vi "GettingHistoricalDataA.vi"() -> ()   [LabVIEW 2020]
uses:
  StateH.ctl
  Data2.ctl
  <vilib>/Utility/file.llb/Read Delimited Spreadsheet (DBL).vi
panel:
  out "StateH":T1=enum."Wait"
  in  "Open Button":bool
  in  "stop":bool
  in  "Play Button":bool
  out "Temperature Graph":T2(graph)
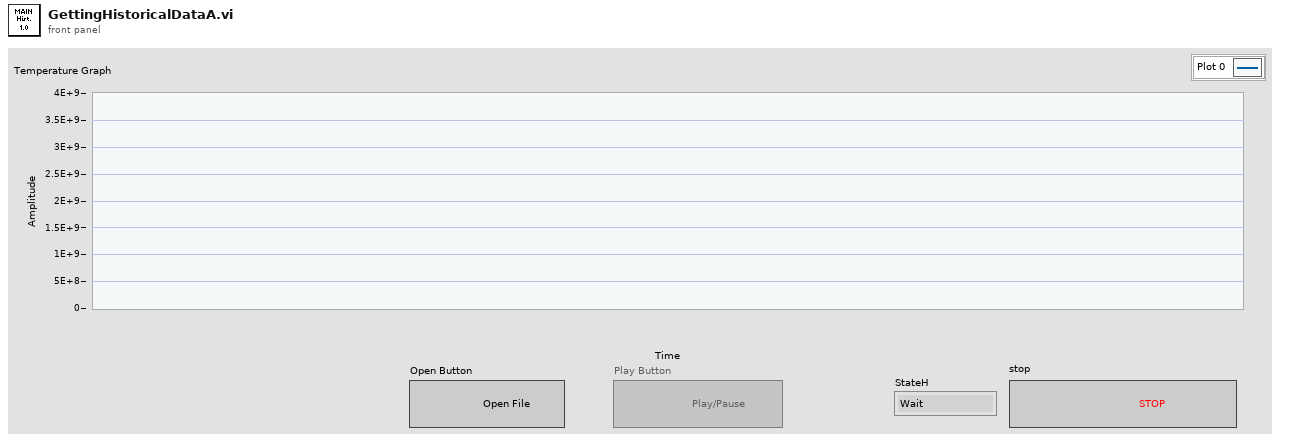
[diagram p1: front panel]
types:
  T1 = typedef "StateH.ctl" = enum16{"Initialize", "Wait", "OpenData", "Play", "Pause", "Finalize"}
  T2 = cluster{"seconds since 1Jan1904":timestamp, dbl, dbl}[]
  T3 = enum8{"Enabled", "Disabled", "Disabled and Grayed Out"}
  T4 = typedef "Data2.ctl" = cluster{"time":timestamp, "Temperature":dbl, "Viscosity":dbl}
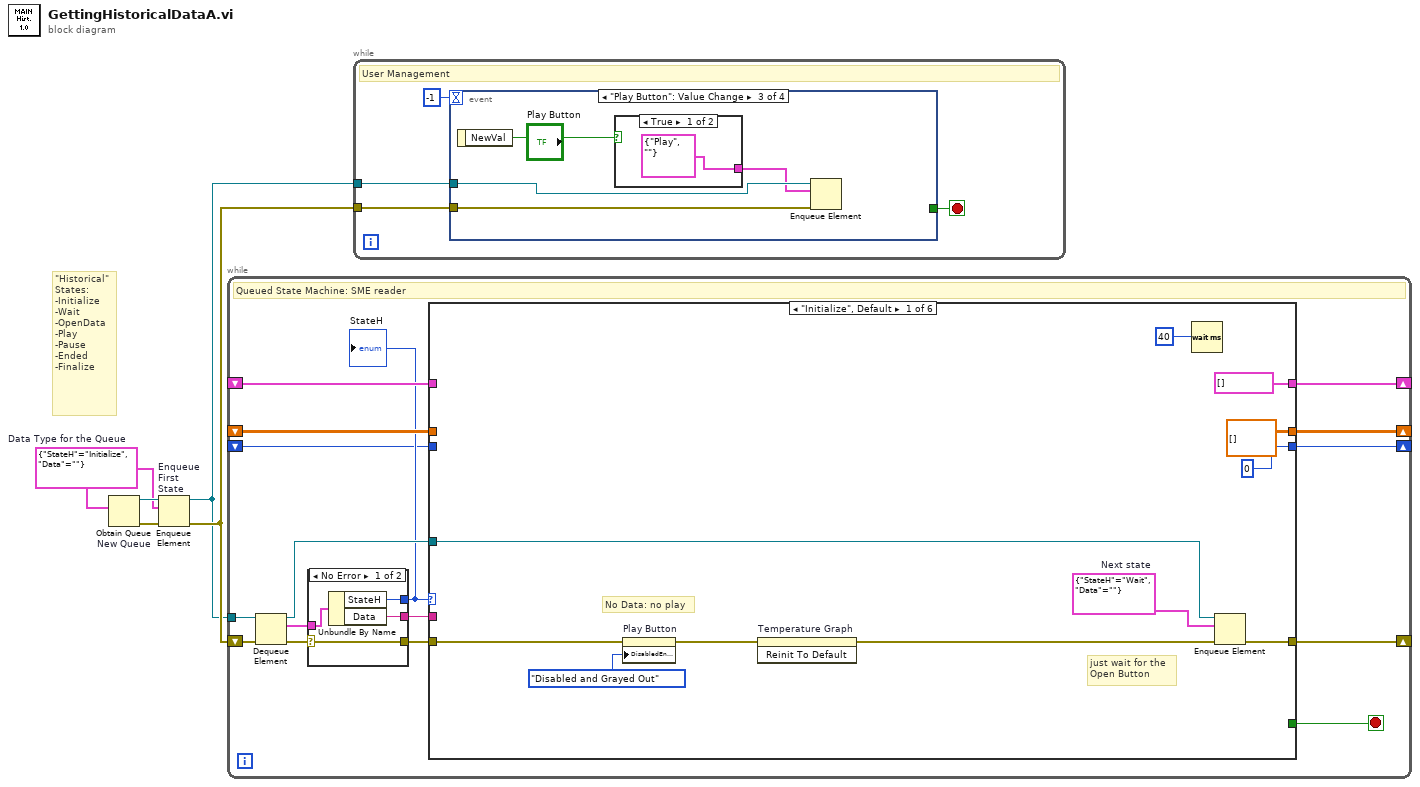
[diagram p0: block diagram]
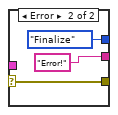
[diagram p2: hidden frame]
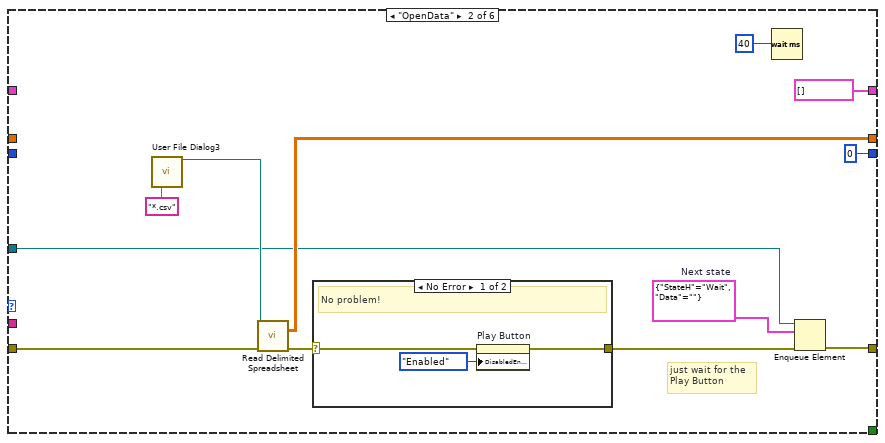
[diagram p3: hidden frame]
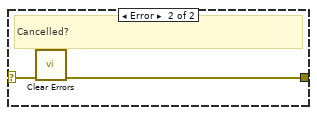
[diagram p4: hidden frame]
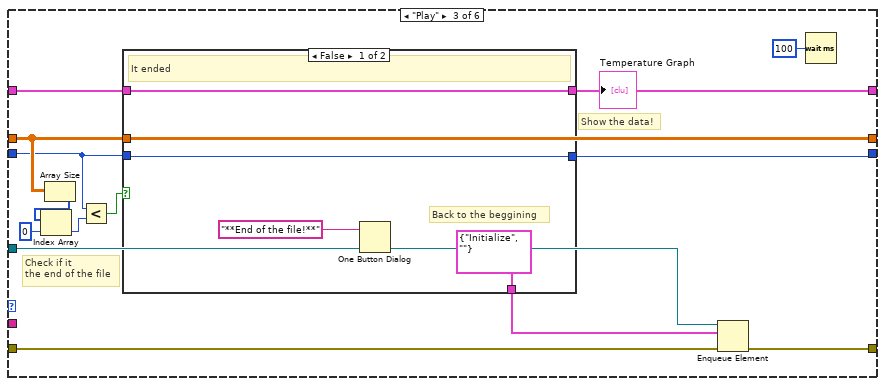
[diagram p5: hidden frame]
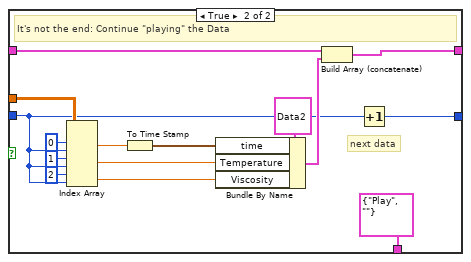
[diagram p6: hidden frame]
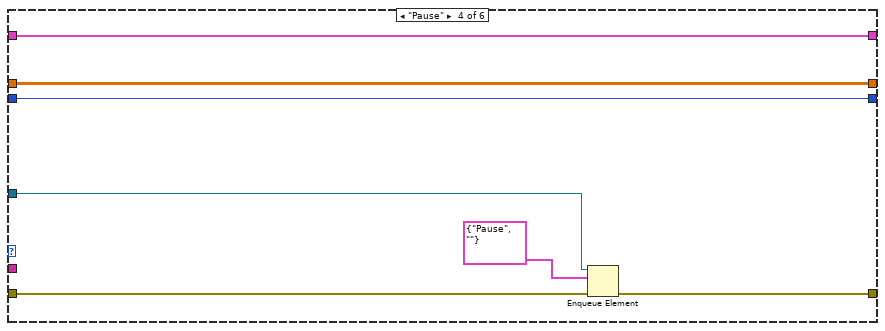
[diagram p7: hidden frame]
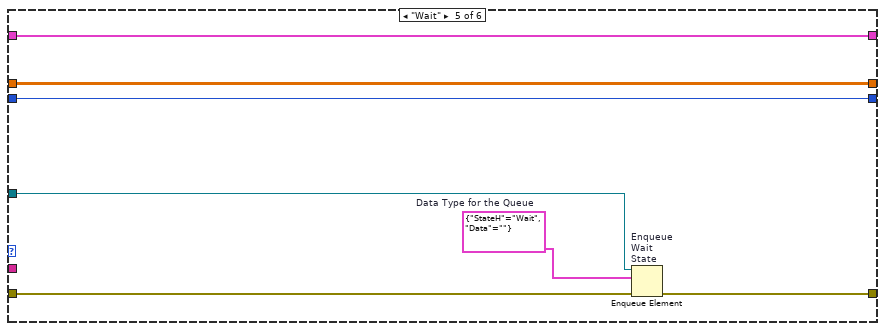
[diagram p8: hidden frame]
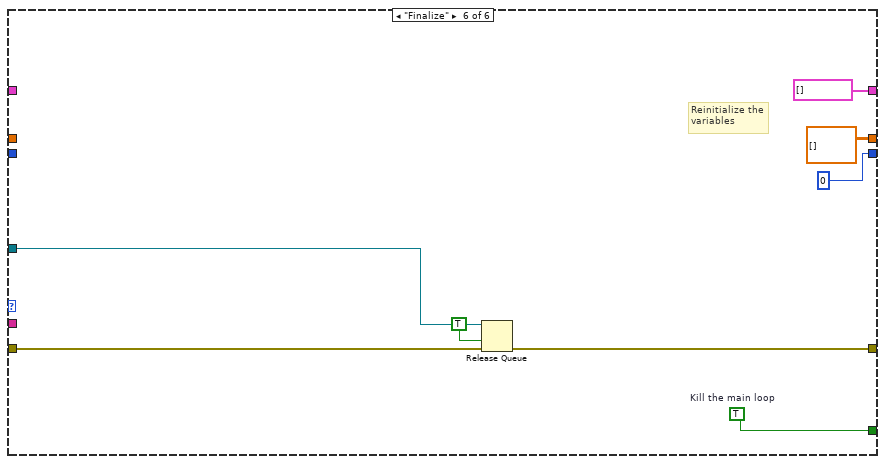
[diagram p9: hidden frame]
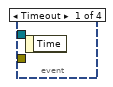
[diagram p10: hidden frame]
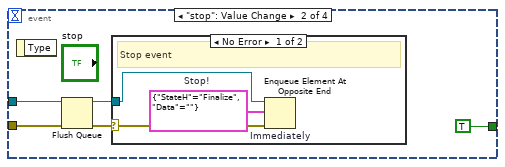
[diagram p11: hidden frame]
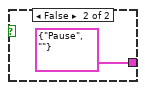
[diagram p13: hidden frame]
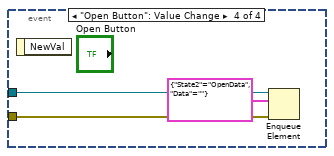
[diagram p14: hidden frame]
diagram:
  w4 = cluster{"StateH":T1, "Data":string} {"StateH"=enum."Initialize", "Data"=""}  # Data Type for the Queue
  # "\"Historical\"\nStates:\n-Initialize\n-Wait\n-OpenData\n-Play\n-Pause\n-Ended\n-Finalize"
  n1 = Obtain Queue "New Queue"(element data type=w4) -> (queue out=w5:refnum<queue>, error out=w3:errorcluster)  [unwired: 4 in, 1 out]
  n2 = Enqueue Element "Enqueue\nFirst\nState"(queue=w5, element=w4, error in (no error)=w3) -> (queue out=w1:refnum<queue>, error out=w2:errorcluster)  [unwired: 1 in, 1 out]
  n3 = while {
    shift-right: [w19] -> _
    shift-left: w2 -> [w18]
    shift-right: [w12] -> _
    shift-left: _ -> [w13]
    shift-right: [w11] -> _
    shift-left: _ -> [w10]
    tunnel: w1 -> [w9]
    shift-right: [w6] -> _
    shift-left: _ -> [w7]
    stop <- w15 stop-if-true
    # "Queued State Machine: SME reader"
    n4 = Dequeue Element(queue=w9, error in (no error)=w18) -> (queue out=w14:refnum<queue>, element=w16:cluster{"StateH":T1, "Data":string}, error out=w17:errorcluster)  [unwired: 1 in, 1 out]
    n5 = case shown="No Error" w17 {
      selector: w17 -> [w22 w27]
      tunnel: w16 -> [w25 _]
      tunnel: [w24 StateH."Finalize" ("StateH")] -> w8
      tunnel: [w23 "Error!" ("Data")] -> w21
      tunnel: [w22 w27] -> w20
      frame No Error {
        n6 = Unbundle By Name(w25) -> ("StateH"=w24:T1, "Data"=w23:string)
      }
      frame Error {
      }
    }
    "StateH" <- w8
    n7 = case shown="\"Initialize\", Default" w8 {
      tunnel: w21 -> [_ _ _ _ _ _]
      tunnel: w20 -> [w33 w41 w67 w90 w99 w106]
      tunnel: [w35 w42 w65 w91 w98 w110] -> w19
      tunnel: [_ _ _ _ _ w111] -> w15
      tunnel: w14 -> [w37 w45 w66 w92 w101 w109]
      tunnel: w13 -> [_ _ w69 w94 w103 _]
      tunnel: [T2 [] T2 [] w68 w94 w103 T2 []] -> w12
      tunnel: [dbl[][] [] ("all rows") w46 w63 w95 w102 dbl[][] [] ("all rows")] -> w11
      tunnel: w10 -> [_ _ w63 w95 w102 _]
      tunnel: w7 -> [_ _ w62 w96 w97 _]
      tunnel: [0 0 w64 w96 w97 0] -> w6
      frame "Initialize", Default {
        w36 = cluster{"StateH":T1, "Data":string} {"StateH"=enum."Wait", "Data"=""}  # Next state
        # "No Data: no play"
        # "just wait for the \nOpen Button"
        n8 = property on="Play Button" class="Bool"(error in=w33, "DisabledEnum"=T3."Disabled and Grayed Out" ("Disabled")) -> (error out=w30:errorcluster)  [unwired: 1 in, 1 out]
        n9 = invoke on="Temperature Graph" class="XYGraph (strict)" method="Reinit To Default"(error in=w30) -> (error out=w29:errorcluster)  [unwired: 2 in, 2 out]
        n10 = Wait (ms)(milliseconds to wait=u32 40) -> ()  [unwired: 1 out]
        n11 = Enqueue Element(queue=w37, element=w36, error in (no error)=w29) -> (error out=w35:errorcluster)  [unwired: 1 in, 2 out]
      }
      frame "OpenData" {
        w44 = cluster{"StateH":T1, "Data":string} {"StateH"=enum."Wait", "Data"=""}  # Next state
        # "just wait for the \nPlay Button"
        n12 = call "User File Dialog3"("pattern (all files)"="*.csv") -> ("selected path"=w47:path)  [unwired: 11 in, 3 out]
        n13 = call-poly <vilib>:"Read Delimited Spreadsheet.vi"("file path (dialog if empty)"=w47, "error in (no error)"=w41) -> ("all rows"=w46:dbl[][], "error out"=w49:errorcluster)  [unwired: 8 in, 4 out]
        n14 = case shown="No Error" w49 {
          selector: w49 -> [w54 w56]
          tunnel: [w53 w55] -> w43
          frame No Error {
            # "No problem!"
            n15 = property on="Play Button" class="Bool"(error in=w54, "DisabledEnum"=T3."Enabled" ("Disabled")) -> (error out=w53:errorcluster)  [unwired: 1 in, 1 out]
          }
          frame Error {
            # "Cancelled?"
            n16 = call <vilib>:"Clear Errors.vi"("error in (no error)"=w56) -> ("error out"=w55:errorcluster)  [unwired: 5 in, 1 out]
          }
        }
        n17 = Wait (ms)(milliseconds to wait=u32 40) -> ()  [unwired: 1 out]
        n18 = Enqueue Element(queue=w45, element=w44, error in (no error)=w43) -> (error out=w42:errorcluster)  [unwired: 1 in, 2 out]
      }
      frame "Play" {
        # "Check if it\nthe end of the file"
        # "Show the data!"
        n19 = Array Size(array=w63) -> (size(s)=w61:i32[])
        n20 = Index Array(array=w61, index=0) -> (element=w59:i32)
        n21 = Less?(x=w62, y=w59) -> (x < y?=w58:bool)
        n22 = case shown="False" w58 {
          tunnel: w69 -> [w74 w89]
          tunnel: [w74 w79] -> w68
          tunnel: w63 -> [_ w78]
          tunnel: w62 -> [w73 w77]
          tunnel: [w73 w76] -> w64
          tunnel: [cluster{"State2":T1, "Data":string} {"State2"=enum."Initialize", "Data"=""} ("element") cluster{"State2":T1, "Data":string} {"State2"=enum."Play", "Data"=""} ("element")] -> w57
          frame False {
            # "Back to the beggining"
            # "It ended"
            n23 = One Button Dialog(message="**End of the file!**") -> ()  [unwired: 1 in, 1 out]
          }
          frame True {
            # "next data"
            # "It's not the end: Continue \"playing\" the Data"
            n24 = Index Array(array=w78, index (row) #1=0 ("index (row)"), index (col) #1=w77, index (row) #2=1 ("disabled index (row)"), index (col) #2=w77, index (row) #3=2 ("disabled index (row)"), index (col) #3=w77) -> (element #1=w85:dbl, element #2=w82:dbl, element #3=w83:dbl)
            n25 = To Time Stamp(1:w85) -> (0:w81:timestamp)
            n26 = Bundle By Name(cluster=T4 {"time"=timestamp(0 s since 1904-01-01), "Temperature"=0.0, "Viscosity"=0.0} ("Data_cluster"), "time"=w81, "Temperature"=w82, "Viscosity"=w83) -> (w80:T4)
            n27 = Build Array (concatenate)(w89, w80) -> (w79:T4[])
            n28 = Increment(x=w77) -> (x+1=w76:i32)
          }
        }
        "Temperature Graph" <- w68
        n29 = Enqueue Element(queue=w66, element=w57, error in (no error)=w67) -> (error out=w65:errorcluster)  [unwired: 1 in, 2 out]
        n30 = Wait (ms)(milliseconds to wait=u32 100) -> ()  [unwired: 1 out]
      }
      frame "Pause" {
        n31 = Enqueue Element(queue=w92, element=cluster{"State2":T1, "Data":string} {"State2"=enum."Pause", "Data"=""}, error in (no error)=w90) -> (error out=w91:errorcluster)  [unwired: 1 in, 2 out]
      }
      frame "Wait" {
        w100 = cluster{"StateH":T1, "Data":string} {"StateH"=enum."Wait", "Data"=""}  # Data Type for the Queue
        n32 = Enqueue Element "Enqueue\nWait\nState"(queue=w101, element=w100, error in (no error)=w99) -> (error out=w98:errorcluster)  [unwired: 1 in, 2 out]
      }
      frame "Finalize" {
        w111 = TRUE  # Kill the main loop
        # "Reinitialize the\nvariables"
        n33 = Release Queue(queue=w109, force destroy? (F)=TRUE, error in (no error)=w106) -> (error out=w110:errorcluster)  [unwired: 2 out]
      }
    }
  }
  n34 = while {
    tunnel: w2 -> [w113]
    tunnel: w1 -> [w112]
    stop <- w114 stop-if-true
    # "User Management"
    n35 = event shown="[2] \"Play Button\": Value Change" {
      selector: _ -> [_ _ _ _]
      dyn-events: _ -> [_ _ _ _]
      timeout: -1 -> [_ _ _ _]
      tunnel: [_ TRUE _ _] -> w114
      tunnel: w113 -> [_ w116 w124 w130]
      tunnel: w112 -> [_ w117 w126 w131]
      event Timeout {
        n36 = event-data() -> ()  [unwired: 1 in, 1 out]
      }
      event "stop": Value Change {
        n37 = event-data() -> ()  [unwired: 1 in, 1 out]
        n38 = Flush Queue(queue=w117, error in (no error)=w116) -> (queue out=w119:refnum<queue>, error out=w118:errorcluster)  [unwired: 1 out]
        n39 = case shown="No Error" w118 {
          selector: w118 -> [w122 _]
          tunnel: w119 -> [w123 _]
          frame No Error {
            w121 = cluster{"StateH":T1, "Data":string} {"StateH"=enum."Finalize", "Data"=""}  # Stop!
            # "Stop event"
            n40 = Enqueue Element At Opposite End "Immediately"(queue=w123, element=w121, error in (no error)=w122) -> ()  [unwired: 1 in, 3 out]
          }
          frame Error {
            # "Already dead"
          }
        }
      }
      event "Play Button": Value Change {
        n41 = event-data() -> ("NewVal"=w127:bool)  [unwired: 1 in]
        n42 = case shown="True" w127 {
          tunnel: [cluster{"State2":T1, "Data":string} {"State2"=enum."Play", "Data"=""} ("element") cluster{"State2":T1, "Data":string} {"State2"=enum."Pause", "Data"=""} ("element")] -> w125
          frame True {
          }
          frame False {
          }
        }
        n43 = Enqueue Element(queue=w126, element=w125, error in (no error)=w124) -> ()  [unwired: 1 in, 3 out]
      }
      event "Open Button": Value Change {
        n44 = event-data() -> ()  [unwired: 1 in, 1 out]
        n45 = Enqueue Element(queue=w131, element=cluster{"State2":T1, "Data":string} {"State2"=enum."OpenData", "Data"=""}, error in (no error)=w130) -> ()  [unwired: 1 in, 3 out]
      }
    }
  }
